vi "Measurement.WavelengthSweeping.TestLauncher.vi"() -> ()   [LabVIEW 2017]
doc: "JKI State Machine Objects (SMO) 1.0.0.5\nJKI - JKI\nCopyright (c) 2016, JKI"
uses:
  Typedefs/Configuration--Cluster.ctl
  Measurement/Typedefs/Measurement.Type--Enum.ctl
  Typedefs/Configuration.Hardware--Cluster.ctl
  Measurement/Typedefs/Configuration.SMU--Cluster.ctl
  SMU/Typedefs/Configuration--Cluster.ctl
  Measurement/Typedefs/Configuration.LIA--Cluster.ctl
  LIA/Typedefs/Configuration--Cluster.ctl
  Measurement/Typedefs/Configuration.OPM--Cluster.ctl
  OPM/Typedefs/Configuration--Cluster.ctl
  Measurement/Typedefs/Configuration.OPA--Cluster.ctl
  OPA/Typedefs/Configuration--Cluster.ctl
  Typedefs/Configuration.Measurement--Cluster.ctl
  Measurement.WavelengthSweeping.lvclass
  D:/Program Files (x86)/National Instruments/LabVIEW 2017/vi.lib/JKI/JKI SMO/SMO/SMO.lvclass
  D:/upwork/Laser Measurement Tool/Laser/project/Subsystems/Measurement/Measurement.lvclass
  Measurement.WavelengthSweeping.UI/Measurement.WavelengthSweeping.UI.lvclass
  D:/upwork/Laser Measurement Tool/Laser/project/Subsystems/Measurement.UI/Measurement.UI.lvclass
  D:/Program Files (x86)/National Instruments/LabVIEW 2017/vi.lib/JKI/JKI SMO/SMO.UI/SMO.UI.lvclass
  <vilib>/JKI/JKI SMO/SMO/SMO.lvclass
  <vilib>/Utility/config.llb/NI_LVConfig.lvlib
  Measurement/Measurement.lvclass
  SMU/SMU.lvclass
  LIA/LIA.lvclass
  OPM/OPM.lvclass
  OPA/OPA.lvclass
  <vilib>/JKI/JKI SMO/SMO.UI/SMO.UI.lvclass
  Measurement.UI/Measurement.UI.lvclass
panel:
  in  "Configuration File Switch":bool=TRUE
  in  "Stop":bool
  # "Measurement.WavelengthSweeping Test Launcher"
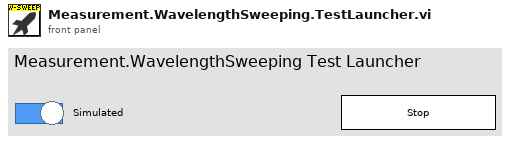
[diagram p1: front panel]
types:
  T1 = typedef "Measurement.WavelengthSweeping.lvclass/Configuration--Cluster.ctl" = cluster{"Measurement.Type":T2, "Hardware":T3, "Measurement":T12}
  T2 = typedef "Measurement.lvclass/Measurement.Type--Enum.ctl" = enum16{"Free", "I/V Curve", "Wavelength sweeping", "Photocurrent mapping"}
  T3 = typedef "Measurement.WavelengthSweeping.lvclass/Configuration.Hardware--Cluster.ctl" = cluster{"SMU":T4, "LIA":T6, "OPM":T8, "OPA":T10}
  T4 = typedef "Measurement.lvclass/Configuration.SMU--Cluster.ctl" = cluster{"Enable":bool, "SMU Model":string, "Configuration":T5}
  T5 = typedef "SMU.lvclass/Configuration--Cluster.ctl" = cluster{"VISA Resource":string, "Channel":string}
  T6 = typedef "Measurement.lvclass/Configuration.LIA--Cluster.ctl" = cluster{"Enable":bool, "LIA Model":string, "Configuration":T7}
  T7 = typedef "LIA.lvclass/Configuration--Cluster.ctl" = cluster{"VISA Resource":string}
  T8 = typedef "Measurement.lvclass/Configuration.OPM--Cluster.ctl" = cluster{"Enable":bool, "OPM Model":string, "Configuration":T9}
  T9 = typedef "OPM.lvclass/Configuration--Cluster.ctl" = cluster{"VISA Resource":string}
  T10 = typedef "Measurement.lvclass/Configuration.OPA--Cluster.ctl" = cluster{"Enable":bool, "OPA Model":string, "Configuration":T11}
  T11 = typedef "OPA.lvclass/Configuration--Cluster.ctl" = cluster{"Serial Number":string}
  T12 = typedef "Measurement.WavelengthSweeping.lvclass/Configuration.Measurement--Cluster.ctl" = cluster{"SMU Voltage, V":dbl, "OPA Start wavelength, nm":dbl, "OPA Stop wavelength, nm":dbl, "OPA Scan resolution, nm":dbl, "OPA Number or points":u16, "Integration time, sec":dbl, "Delay time, ms":u16, "Accumulation":u16}
  T13 = typedef "NI_LVConfig.lvlib/Config Data RefNum.ctl" = refnum<k1>
  T14 = typedef "SMO.lvclass/Public Events.ctl" = cluster{"Error":refnum<user-event>, "State":refnum<user-event>, "Reserve State":refnum<user-event>}
  T15 = cluster{"SMO.UI Public Events":refnum<event-registration>, "Event Registration Refnum":refnum<event-registration>}
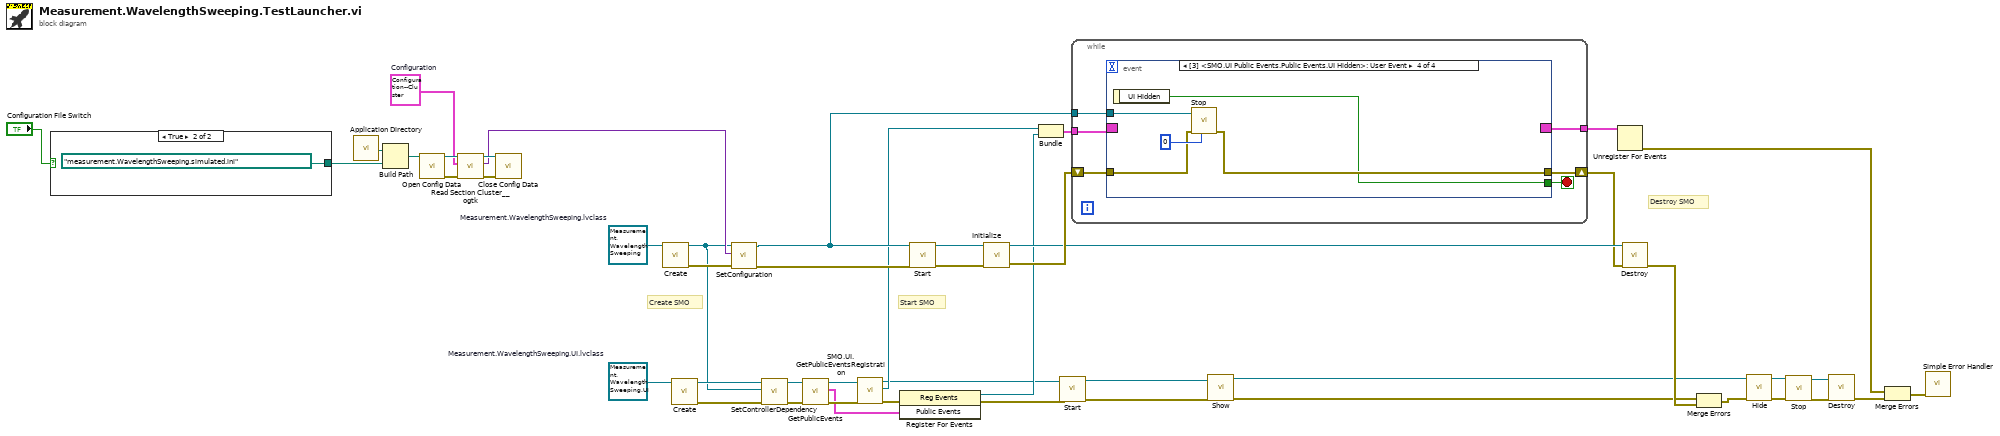
[diagram p0: block diagram]
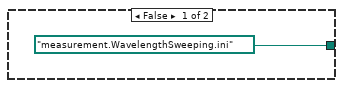
[diagram p2: hidden frame]
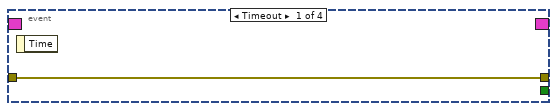
[diagram p3: hidden frame]
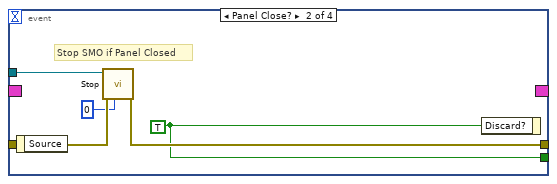
[diagram p4: hidden frame]
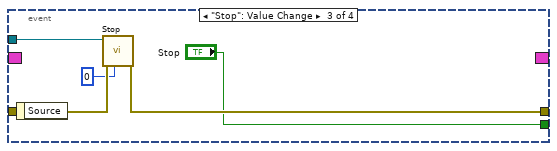
[diagram p5: hidden frame]
diagram:
  w29 = refnum<class "Measurement.WavelengthSweeping.UI.lvclass"> refnum  # Measurement.WavelengthSweeping.UI.lvclass
  w37 = refnum<class "Measurement.WavelengthSweeping.lvclass"> refnum  # Measurement.WavelengthSweeping.lvclass
  w38 = T1 {"Measurement.Type"=enum."Wavelength sweeping", "Hardware"={"SMU"={"Enable"=FALSE, "SMU Model"="", "Configuration"={"VISA Resource"="", "Channel"=""}}, "LIA"={"Enable"=FALSE, "LIA Model"="", "Configuration"={"VISA Resource"=""}}, "OPM"={"Enable"=FALSE, "OPM Model"="", "Configuration"={"VISA Resource"=""}}, "OPA"={"Enable"=FALSE, "OPA Model"="", "Configuration"={"Serial Number"=""}}}, "Measurement"={"SMU Voltage, V"=0.0, "OPA Start wavelength, nm"=0.0, "OPA Stop wavelength, nm"=0.0, "OPA Scan resolution, nm"=0.0, "OPA Number or points"=0, "Integration time, sec"=0.0, "Delay time, ms"=0, "Accumulation"=0}}  # Configuration
  # "Start SMO"
  # "Destroy SMO"
  # "Create SMO"
  n1 = case shown="True" "Configuration File Switch" {
    tunnel: [path "measurement.WavelengthSweeping.ini" path "measurement.WavelengthSweeping.simulated.ini"] -> w39
    frame False {
    }
    frame True {
    }
  }
  n2 = call <vilib>:"Application Directory.vi"() -> ("Application Directory"=w45:path)
  n3 = Build Path(base path=w45, name or relative path=w39) -> (appended path=w44:path)
  n4 = call <vilib>:"Open Config Data.vi"("configuration file path"=w44) -> ("error out"=w43:errorcluster, "refnum"=w42:T13)  [unwired: 8 in, 1 out]
  n5 = call <userlib>:"Read Section Cluster__ogtk.vi"("error in (no error)"=w43, "Section Formatted Cluster Type"=w38, "refnum"=w42) -> ("error out"=w40:errorcluster, "Section Formatted Cluster"=w2:variant, "dup refnum"=w41:T13)  [unwired: 4 in, 2 out]
  n6 = call <vilib>:"Close Config Data.vi"("error in (no error)"=w40, "refnum"=w41) -> ()  [unwired: 8 in, 2 out]
  n7 = call <vilib>:"Create.vi"("SMO"=w37) -> ("error out"=w36:errorcluster, "SMO out"=w1:refnum<class "Measurement.WavelengthSweeping.lvclass">)  [unwired: 8 in, 1 out]
  n8 = call <vilib>:"Create.vi"("SMO"=w29) -> ("error out"=w27:errorcluster, "SMO out"=w28:refnum<class "Measurement.WavelengthSweeping.UI.lvclass">)  [unwired: 8 in, 1 out]
  n9 = call "SetConfiguration.vi"("error in (no error)"=w36, "Configuration"=w2, "Measurement in"=w1) -> ("error out"=w34:errorcluster, "Measurement out"=w35:refnum<class "Measurement.WavelengthSweeping.lvclass">)  [unwired: 7 in]
  n10 = call "SetControllerDependency.vi"("error in (no error)"=w27, "Measurement"=w1, "Measurement.UI in"=w28) -> ("error out"=w23:errorcluster, "Measurement.UI out"=w24:refnum<class "Measurement.WavelengthSweeping.UI.lvclass">)  [unwired: 7 in]
  n11 = call <vilib>:"GetPublicEvents.vi"("error in (no error)"=w23, "SMO"=w24) -> ("error out"=w26:errorcluster, "Public Events"=w22:T14, "SMO out"=w25:refnum<class "Measurement.WavelengthSweeping.UI.lvclass">)  [unwired: 7 in]
  n12 = call <vilib>:"SMO.UI.GetPublicEventsRegistration.vi"("error in (no error)"=w26, "SMO.UI"=w25) -> ("error out"=w21:errorcluster, "SMO.UI Public Events"=w19:refnum<event-registration>, "SMO.UI out"=w17:refnum<class "Measurement.WavelengthSweeping.UI.lvclass">)  [unwired: 7 in]
  n13 = register-events(error in=w21, w22) -> (reference out=w18:refnum<event-registration>, error out=w16:errorcluster)  [unwired: 1 in]
  n14 = call <vilib>:"Start.vi"("error in (no error)"=w34, "SMO"=w35) -> ("error out"=w32:errorcluster, "SMO out"=w33:refnum<class "Measurement.WavelengthSweeping.lvclass">)  [unwired: 8 in]
  n15 = call "Initialize.vi"("error in (no error)"=w32, "Measurement in"=w33) -> ("error out"=w31:errorcluster, "Measurement out"=w30:refnum<class "Measurement.WavelengthSweeping.lvclass">)  [unwired: 8 in]
  n16 = Bundle("SMO.UI Public Events"=w19, "Event Registration Refnum"=w18) -> (w20:T15)  [unwired: 1 in]
  n17 = call <vilib>:"Start.vi"("error in (no error)"=w16, "SMO"=w17) -> ("error out"=w14:errorcluster, "SMO out"=w15:refnum<class "Measurement.WavelengthSweeping.UI.lvclass">)  [unwired: 8 in]
  n18 = while {
    shift-right: [w55] -> w13
    shift-left: w31 -> [w54]
    tunnel: [w53] -> w48
    tunnel: w35 -> [w52]
    tunnel: w20 -> [w51]
    stop <- w56 stop-if-true
    n19 = event shown="[3] <SMO.UI Public Events.Public Events.UI Hidden>: User Event" {
      selector: w51 -> [_ _ _ _]
      dyn-events: [_ _ _ _] -> w53
      timeout: _ -> [_ _ _ _]
      tunnel: [_ w59 "Stop" w68] -> w56
      tunnel: w52 -> [_ w62 w67 w71]
      tunnel: [w57 w61 w66 w69] -> w55
      tunnel: w54 -> [w57 w60 w65 w70]
      event Timeout {
        n20 = event-data() -> ()  [unwired: 1 in, 1 out]
      }
      event Panel Close? {
        w59 = TRUE ("OK")
        # "Stop SMO if Panel Closed"
        n21 = event-data() -> ()  [unwired: 1 in, 1 out]
        n22 = call <vilib>:"Stop.vi"("timeout in ms (-1)"=0, "error in (no error)"=w60, "SMO"=w62) -> ("error out"=w61:errorcluster)  [unwired: 7 in, 1 out]
        n23 = event-data("Discard?"=w59) -> ()  [unwired: 1 in, 1 out]
      }
      event "Stop": Value Change {
        n24 = event-data() -> ()  [unwired: 1 in, 1 out]
        n25 = call <vilib>:"Stop.vi"("timeout in ms (-1)"=0, "error in (no error)"=w65, "SMO"=w67) -> ("error out"=w66:errorcluster)  [unwired: 7 in, 1 out]
      }
      event User Event {
        n26 = event-data() -> ("UI Hidden"=w68:bool)  [unwired: 1 in]
        n27 = call <vilib>:"Stop.vi"("timeout in ms (-1)"=0, "error in (no error)"=w70, "SMO"=w71) -> ("error out"=w69:errorcluster)  [unwired: 7 in, 1 out]
      }
    }
  }
  n28 = call <vilib>:"Show.vi"("error in (no error)"=w14, "SMO.UI"=w15) -> ("error out"=w12:errorcluster, "SMO.UI out"=w7:refnum<class "Measurement.WavelengthSweeping.UI.lvclass">)  [unwired: 8 in]
  n29 = Unregister For Events(event registration refnum=w48) -> (error out=w3:errorcluster)  [unwired: 1 in]
  n30 = call <vilib>:"Destroy.vi"("error in (no error)"=w13, "SMO"=w30) -> ("error out"=w47:errorcluster)  [unwired: 9 in]
  n31 = Merge Errors(w12, w47) -> (w6:errorcluster)
  n32 = call <vilib>:"Hide.vi"("error in (no error)"=w6, "SMO.UI"=w7) -> ("error out"=w9:errorcluster, "SMO.UI out"=w8:refnum<class "Measurement.WavelengthSweeping.UI.lvclass">)  [unwired: 8 in]
  n33 = call <vilib>:"Stop.vi"("error in (no error)"=w9, "SMO"=w8) -> ("error out"=w10:errorcluster, "SMO out"=w11:refnum<class "Measurement.WavelengthSweeping.UI.lvclass">)  [unwired: 8 in]
  n34 = call <vilib>:"Destroy.vi"("error in (no error)"=w10, "SMO"=w11) -> ("error out"=w4:errorcluster)  [unwired: 9 in]
  n35 = Merge Errors(w3, w4) -> (w5:errorcluster)
  n36 = call <vilib>:"Simple Error Handler.vi"("error in (no error)"=w5) -> ()  [unwired: 4 in, 5 out]
